vi "API Initialize.vi"(8 "error in (no error)":errorcluster, 9 "Temperature Lower Limit":dbl min=-200.0 max=300.0 step=1.0 format="%.1f", 10 "Temperature Upper Limit":dbl min=-200.0 max=300.0 step=1.0 format="%.1f", 11 "VISA resource name":refnum<visa-resource-name>="TCPIP::127.0.0.1::8888::SOCKET") -> (0 "error out":errorcluster, 3 "VISA resource out":refnum<visa-resource-name>)   [LabVIEW 2024, in "Thermotron 8800.lvlib"]
uses:
  Thermotron 8800.lvlib
  Private/OptionWordSelection.ctl
  Private/get set.ctl
  Private/AnalogInputChannelNumber 1-4.ctl
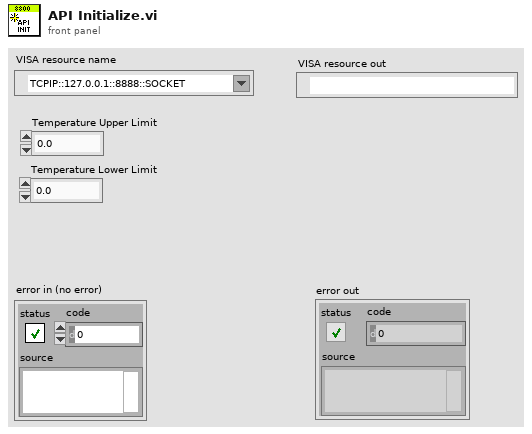
[diagram p1: front panel]
types:
  T1 = typedef "Thermotron 8800.lvlib/AnalogInputChannelNumber 1-4.ctl" = u16
  T2 = typedef "Thermotron 8800.lvlib/get set.ctl" = enum16{"get", "set"}
  T3 = typedef "Thermotron 8800.lvlib/OptionWordSelection.ctl" = u16
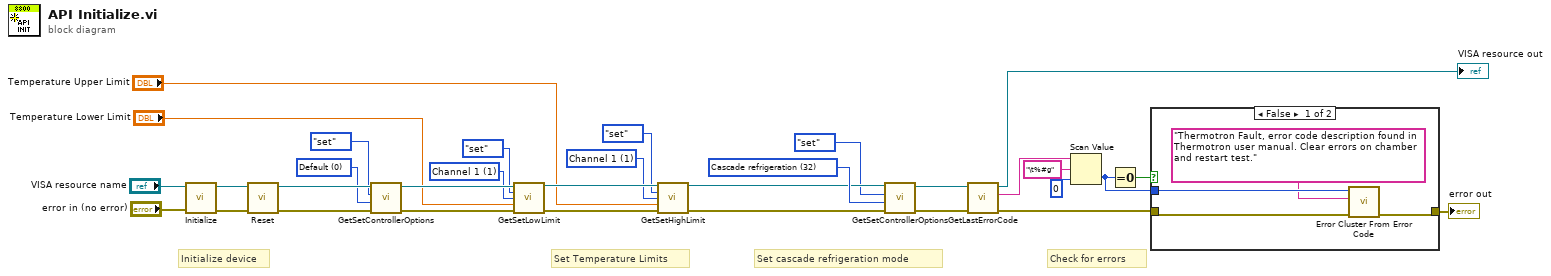
[diagram p0: block diagram]
diagram:
  w4 = T1 1 items=["Channel 1"=1, "Channel 2"=2, "Channel 3"=3, "Channel 4"=4] ("Channel Number (1-4)")
  w7 = T1 1 items=["Channel 1"=1, "Channel 2"=2, "Channel 3"=3, "Channel 4"=4] ("Channel Number (1-4)")
  w11 = T3 0 items=["Default"=0, "Product temperature control"=1, "Humidity system"=2, "Low humidity system"=4, "GSoak"=8, "Purge"=16, "Cascade refrigeration"=32, "Power Save mode"=64, "Single-stage refrig."=128, "Altitude"=512, "Mechanical boost"=1024, "Product dewpoint control"=32768] ("Option (may be added for multiple)")
  w32 = T3 32 items=["Product temperature control"=1, "Humidity system"=2, "Low humidity system"=4, "GSoak"=8, "Purge"=16, "Cascade refrigeration"=32, "Power Save mode"=64, "Single-stage refrig."=128, "Altitude"=512, "Mechanical boost"=1024, "Product dewpoint control"=32768] ("Option (may be added for multiple)")
  # "Check for errors"
  # "Set cascade refrigeration mode"
  # "Set Temperature Limits"
  # "Initialize device"
  n1 = call "Initialize.vi"("error in (no error)"="error in (no error)", "VISA resource name"="VISA resource name") -> ("error out"=w29:errorcluster, "VISA resource name out"=w30:refnum<visa-resource-name>)  [unwired: 7 in, 1 out]
  n2 = call "Reset.vi"("error in (no error)"=w29, "VISA resource name"=w30) -> ("error out"=w27:errorcluster, "VISA resource name out"=w28:refnum<visa-resource-name>)  [unwired: 8 in]
  n3 = call "GetSetControllerOptions.vi"("error in"=w27, "Option (may be added for multiple)"=w11, "get/set"=get_set."set", "VISA resource name"=w28) -> ("error out"=w25:errorcluster, "VISA resource name out"=w26:refnum<visa-resource-name>)  [unwired: 5 in, 1 out]
  n4 = call "GetSetLowLimit.vi"("VISA resource name"=w26, "get/set"=get_set."set", "Channel Number (1-4)"=w7, "Setpoint"="Temperature Lower Limit", "error in"=w25) -> ("VISA resource name out"=w23:refnum<visa-resource-name>, "error out"=w24:errorcluster)  [unwired: 7 in, 2 out]
  n5 = call "GetSetHighLimit.vi"("VISA resource name"=w23, "get/set"=get_set."set", "Channel Number (1-4)"=w4, "Setpoint"="Temperature Upper Limit", "error in"=w24) -> ("VISA resource name out"=w22:refnum<visa-resource-name>, "error out"=w21:errorcluster)  [unwired: 7 in, 2 out]
  n6 = call "GetSetControllerOptions.vi"("error in"=w21, "Option (may be added for multiple)"=w32, "get/set"=get_set."set", "VISA resource name"=w22) -> ("error out"=w20:errorcluster, "VISA resource name out"=w18:refnum<visa-resource-name>)  [unwired: 5 in, 1 out]
  n7 = call "GetLastErrorCode.vi"("error in"=w20, "VISA resource name"=w18) -> ("error out"=w17:errorcluster, "Last error code"=w14:string, "VISA resource name out"=→"VISA resource out":refnum<visa-resource-name>)  [unwired: 6 in, 1 out]
  n8 = Scan Value(string=w14, format string="\t%#g", default (0 dbl)=0) -> (value=w13:i32)  [unwired: 1 out]
  n9 = Equal To 0?(x=w13) -> (x = 0?=w31:bool)
  n10 = case shown="False" w31 {
    tunnel: w17 -> [w36 w37]
    tunnel: w13 -> [w35 _]
    tunnel: [w34 w37] -> w2
    frame False {
      n11 = call <vilib>:"Error Cluster From Error Code.vi"("error in (no error)"=w36, "error message (\"\")"="Thermotron Fault, error code description found in Thermotron user manual. Clear errors on chamber and restart test." ("error message (\"\")"), "error code (0)"=w35) -> ("error out"=w34:errorcluster)  [unwired: 6 in]
    }
    frame True {
    }
  }
  "error out" <- w2
